vi "Dynamic Load and Execute Tests Process.vi"(7 "API_TextTestRunner":refnum<class>, 8 "error in":errorcluster, 9 "App Data":T1, 10 "Operation":enum16{"Load", "Run Test", "Run All Tests"}(ring), 11 "Test Hierarchy Tree":refnum<vi>) -> (0 "error out":errorcluster, 1 "Tree Methods":i32)   [LabVIEW 2011, in "GraphicalTestRunner.lvlib"]
uses:
  GraphicalTestRunner.lvlib
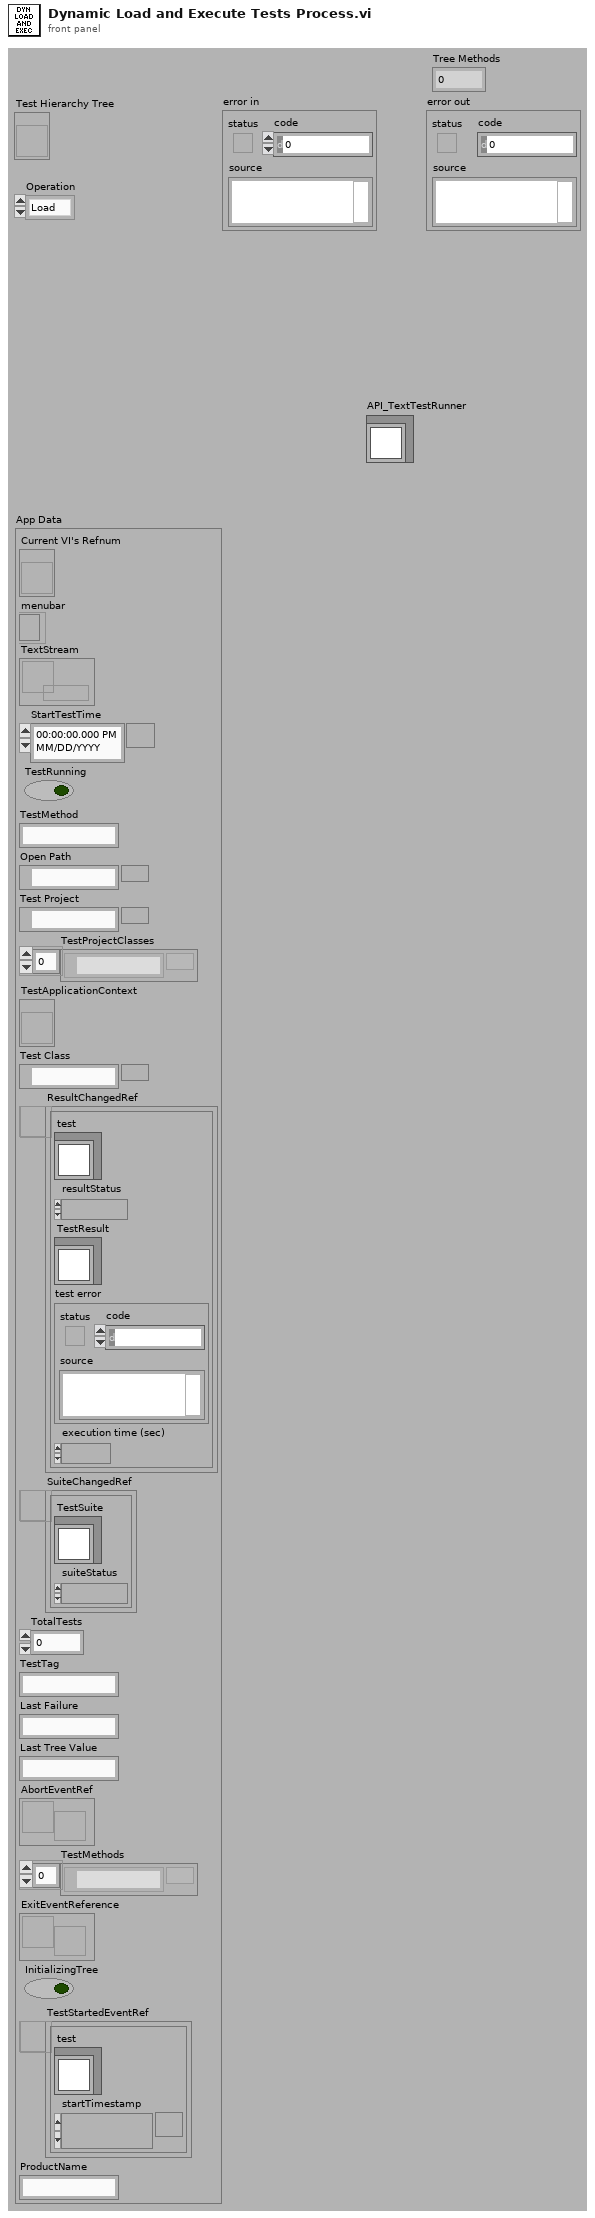
[diagram p1: front panel]
types:
  T1 = cluster{"Current VI's Refnum":refnum<vi>, "menubar":refnum<k9>, "TextStream":refnum<queue>, "StartTestTime":timestamp, "TestRunning":bool, "TestMethod":string, "Open Path":path, "Test Project":path, "TestProjectClasses":path[], "TestApplicationContext":refnum<vi>, "Test Class":path, "ResultChangedRef":refnum<user-event>, "SuiteChangedRef":refnum<user-event>, "TotalTests":i32, "TestTag":string, "Last Failure":string, "Last Tree Value":string, "AbortEventRef":refnum<user-event>, "TestMethods":path[], "ExitEventReference":refnum<user-event>, "InitializingTree":bool, "TestStartedEventRef":refnum<user-event>, "ProductName":string}
  T2 = cluster{"ResultStatusChanged":refnum<user-event>, "SuiteStatusChanged":refnum<user-event>, "Exit":refnum<user-event>, "TestStartedEventRef":refnum<user-event>}
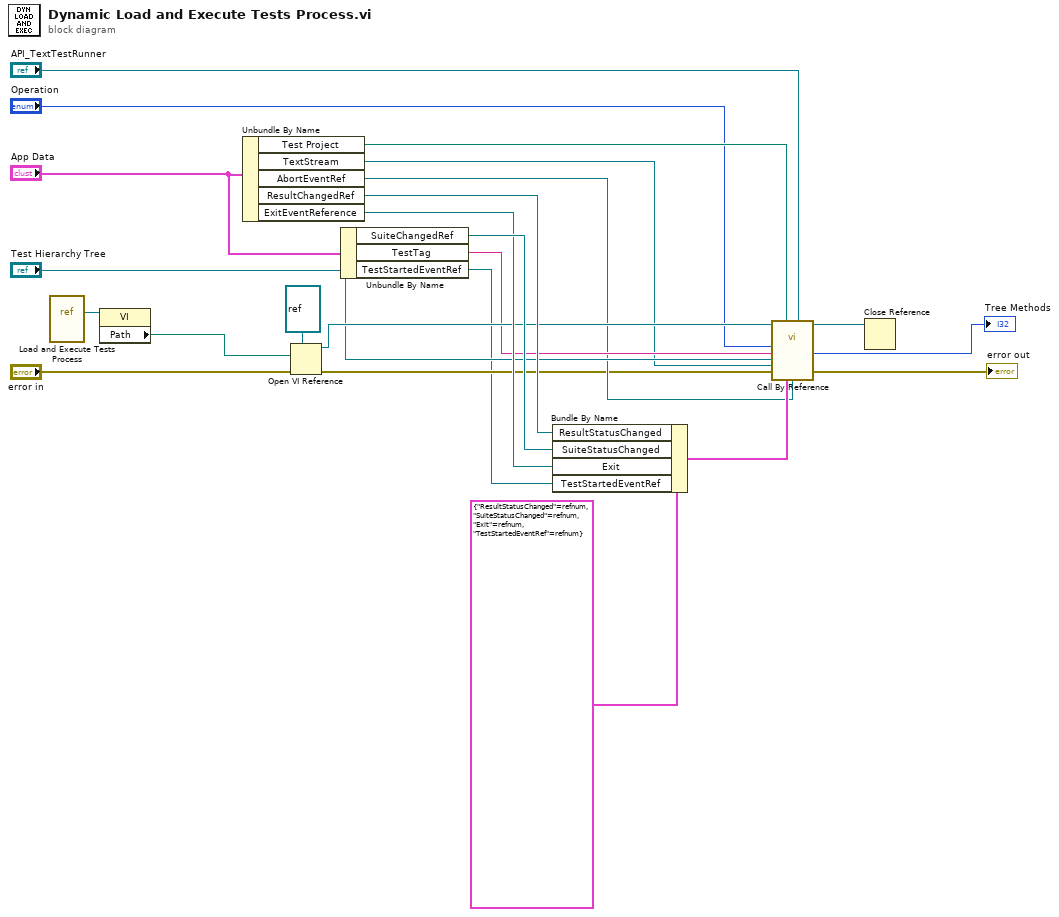
[diagram p0: block diagram]
diagram:
  n1 = vi-ref "Load and Execute Tests Process.vi"() -> (w1:refnum<vi>)
  n2 = property class="VI"(reference=w1) -> ("Path"=w17:path)  [unwired: 1 in, 2 out]
  n3 = Unbundle By Name("App Data") -> ("Test Project"=w16:path, "TextStream"=w12:refnum<queue>, "AbortEventRef"=w10:refnum<user-event>, "ResultChangedRef"=w20:refnum<user-event>, "ExitEventReference"=w19:refnum<user-event>)
  n4 = Open VI Reference(type specifier VI Refnum (for type only)=refnum<vi> refnum, vi path=w17, error in (no error)="error in") -> (vi reference=w18:refnum<vi>, error out=w7:errorcluster)  [unwired: 3 in]
  n5 = Unbundle By Name("App Data") -> ("SuiteChangedRef"=w22:refnum<user-event>, "TestTag"=w14:string, "TestStartedEventRef"=w2:refnum<user-event>)
  n6 = Bundle By Name(cluster=T2 {"ResultStatusChanged"=refnum, "SuiteStatusChanged"=refnum, "Exit"=refnum, "TestStartedEventRef"=refnum} ("TestStatusEvents"), "ResultStatusChanged"=w20, "SuiteStatusChanged"=w22, "Exit"=w19, "TestStartedEventRef"=w2) -> (w11:T2)
  n7 = call-by-ref "?"(reference=w18, "Operation"="Operation", "Test Project"=w16, "API_TextTestRunner"="API_TextTestRunner", "TestTag Argument"=w14, "Test Hierarchy Tree ref"="Test Hierarchy Tree", "TextStream"=w12, "error in"=w7, "TestStatusEvents"=w11, "AbortEvent"=w10) -> (reference out=w6:refnum<vi>, "Tree Methods"=→"Tree Methods":i32, "error out"=→"error out":errorcluster)  [unwired: 6 in, 1 out]
  n8 = Close Reference(reference=w6) -> ()  [unwired: 1 in, 1 out]
